vi "FlatToRichexternal_driver_wrapper_InitializeResponse.vi"(5 "OutputClusterType":T1, 11 "InputCluster":T2) -> (3 "OutputCluster":T1)   [LabVIEW 2020, in "Instrument Interaction Client.lvlib"]
uses:
  Instrument Interaction Client.lvlib
  external_driver_wrapper_InitializeResponse_Flat.ctl
  external_driver_wrapper_InitializeResponse.ctl
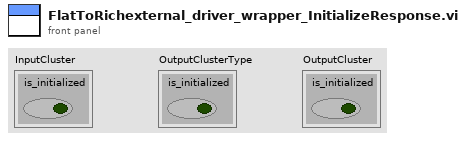
[diagram p1: front panel]
types:
  T1 = typedef "Instrument Interaction Client.lvlib/external_driver_wrapper_InitializeResponse.ctl" = cluster{"is_initialized":bool}
  T2 = typedef "Instrument Interaction Client.lvlib/external_driver_wrapper_InitializeResponse_Flat.ctl" = cluster{"is_initialized":bool}
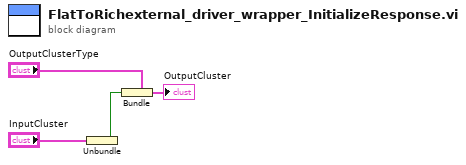
[diagram p0: block diagram]
diagram:
  n1 = Unbundle "Unbundle"("InputCluster") -> ("is_initialized"=w1:bool)
  n2 = Bundle "Bundle"(cluster="OutputClusterType", "is_initialized"=w1) -> (→"OutputCluster":T1)
